vi "Write Pref.vi"() -> (0 "error out":errorcluster)   [LabVIEW 2020, in "Pref Tests.lvlib"]
uses:
  Pref Tests.lvlib
  User Prefs/PrefsDB/PrefsDB.lvclass
  User Prefs/Pref Group/Pref Group.lvclass
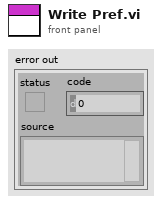
[diagram p1: front panel]
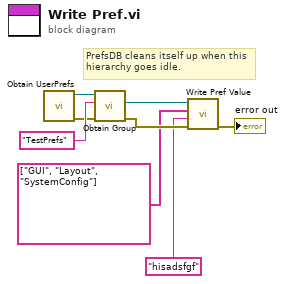
[diagram p0: block diagram]
diagram:
  # "PrefsDB cleans itself up when this hierarchy goes idle."
  n1 = call "Obtain UserPrefs.vi"() -> ("error out"=w2:errorcluster, "PrefsDB out"=w4:refnum<class "PrefsDB.lvclass">)  [unwired: 10 in]
  n2 = call "Obtain Group.vi"("error in (no error)"=w2, "Group"="TestPrefs", "PrefsDB in"=w4) -> ("error out"=w8:errorcluster, "Pref Group"=w1:refnum<class "Pref Group.lvclass">)  [unwired: 6 in, 1 out]
  n3 = call "Write Pref Value.vi"("error in (no error)"=w8, "Value"="hisadsfgf", "Pref Hierarchy"=string[] ["GUI", "Layout", "SystemConfig"], "Pref Group in"=w1) -> ("error out"=→"error out":errorcluster)  [unwired: 6 in, 1 out]
